vi "Interface.vi"(9 "EventsIn":T2, 10 "Events":T3) -> ()   [LabVIEW 2014, in "VIExecutionProperties.lvlib" / "VIExecutionProperties.lvclass"]
uses:
  VIExecutionProperties.lvclass
  Framework/_Plugins/_LVCMPlugin/GCMPlugin_EventsOut.ctl
  Framework/_Plugins/_LVCMPlugin/GCMPlugin_EventsIn.ctl
  Command.ctl
  Framework/_Plugins/GCMPlugin/GCMPlugin.lvclass
panel:
  out "LastCompiledWith":string caption="Last Compiled With:"
  out "CompiledCodeComplexity":dbl caption="Compiled Code Complexity:" format="%.0g"
  out "CodeSize":dbl caption="Code:" format="%01.1f kB"
  out "DataSize":dbl caption="Data:" format="%01.1f kB"
  out "BlockDiagramSize":dbl caption="Block Diagram:" format="%01.1f kB"
  out "FrontPanelSize":dbl caption="Front Panel:" format="%01.1f kB"
  in  "SuspendWhenCalled":bool caption="Suspend when called"
  in  "RunOnOpen":bool caption="Run when opened"
  in  "AutoErrHandling":bool caption="Enable auto error handling"
  in  "Priority":u16(ring) items=["invalid priority", "background", "normal", "above normal", "high", "time critical", "subroutine"]
  in  "PrefferedExecSystem":u16(ring) caption="Preffered execution system" items=["invalid execution system", "user interface", "standard", "instrument i/o", "data acquisition", "other 1", "other 2", "same as caller"]
  in  "Reentrancy":T1(radio)
  in  "InlineSubVI":bool caption="Inline subVI into calling VIs"
  in  "AllowDebugging":bool caption="Allow Debugging"
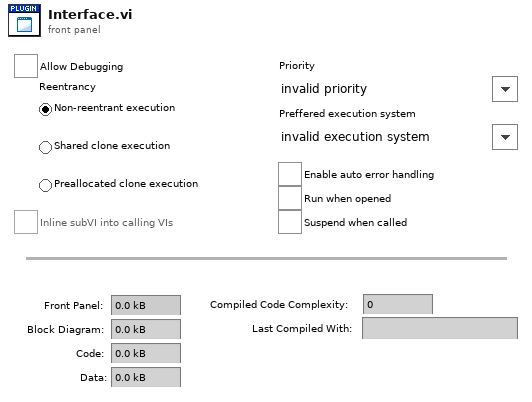
[diagram p1: front panel]
types:
  T1 = enum32{"Non-reentrant", "Shared clone", "Preallocated clone"}
  T2 = typedef "GCMPlugin.lvclass/GCMPlugin_EventsIn.ctl" = cluster{"Stop":refnum<user-event>, "ItemSelected":refnum<user-event>, "ItemDeselected":refnum<user-event>, "PluginActivated":refnum<user-event>, "PluginDeactivated":refnum<user-event>}
  T3 = typedef "GCMPlugin.lvclass/GCMPlugin_EventsOut.ctl" = cluster{"ItemEdited":refnum<user-event>}
  T4 = enum16{"Share clones between instances", "Preallocate clone for each instance"}
  T5 = enum8{"Enabled", "Disabled", "Disabled and Grayed Out"}
  T6 = typedef "VIExecutionProperties.lvlib/VIExecutionProperties.lvclass/Command.ctl" = enum16{"SaveVI", "LoadVIProperties", "Stop"}
  T7 = enum32{"invalid execution system", "user interface", "standard", "instrument i/o", "data acquisition", "other 1", "other 2", "same as caller"}
  T8 = enum32{"invalid priority", "background priority", "normal priority", "above normal priority", "high priority", "time critical priority", "subroutine"}
  T9 = typedef "LVLastCompiledWithTypeDef.ctl" = enum16{"Partial compiler optimizations", "Full compiler optimizations"}
  T10 = cluster{"Metric.FPSize":u32, "Metric.BDSize":u32, "Metric.CodeSize":u32, "Metric.DataSize":u32}
  T11 = cluster{"Metric.FPSize":dbl, "Metric.BDSize":dbl, "Metric.CodeSize":dbl, "Metric.DataSize":dbl}
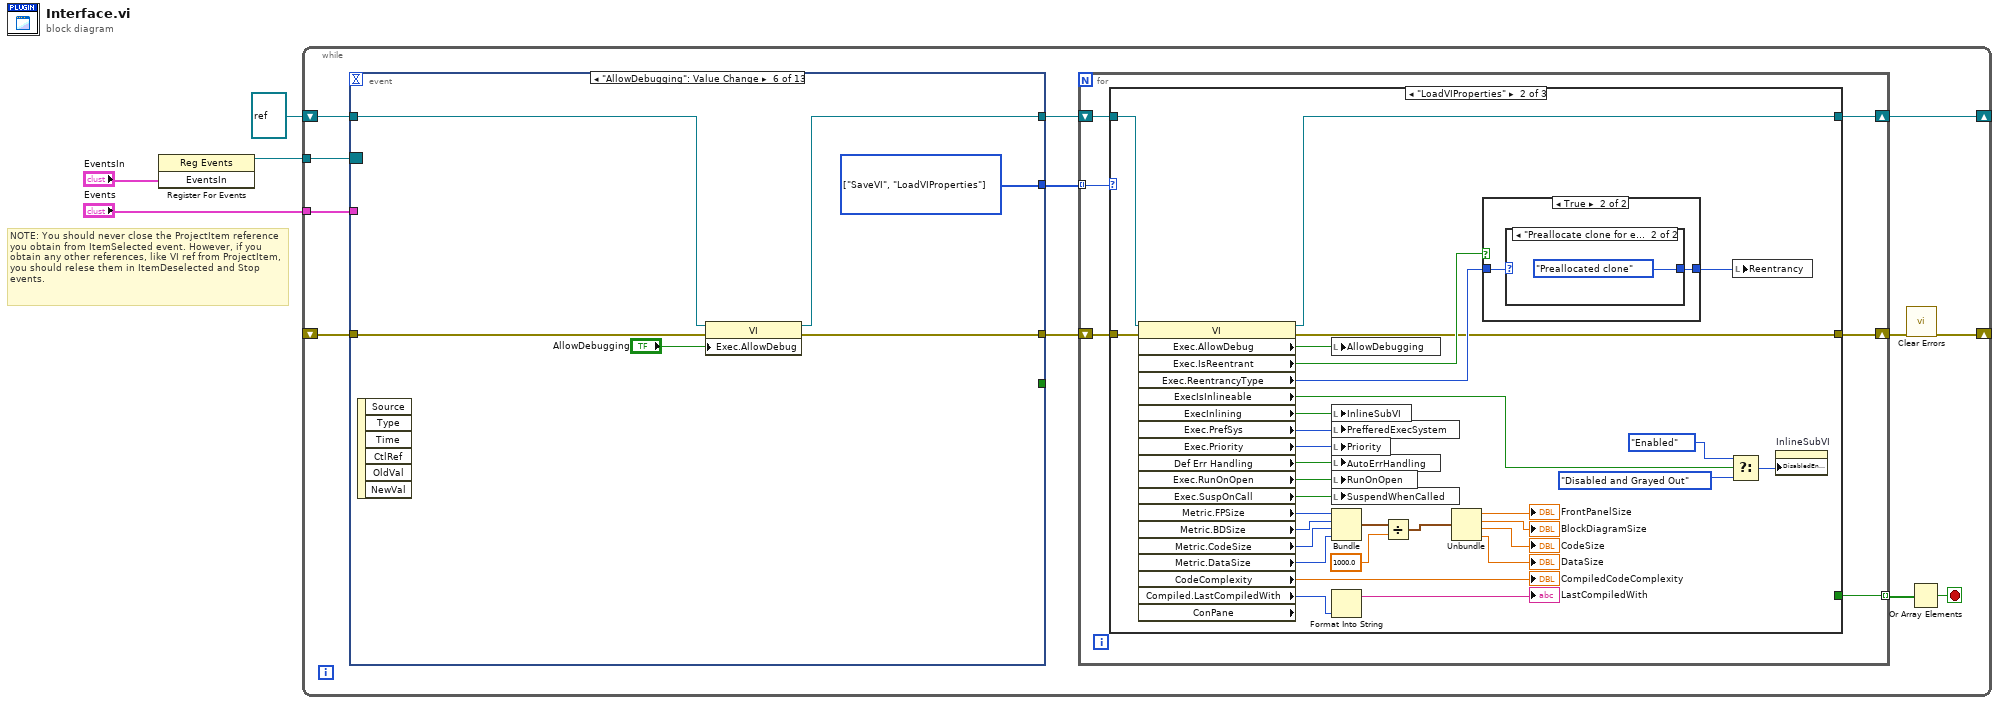
[diagram p0: block diagram]
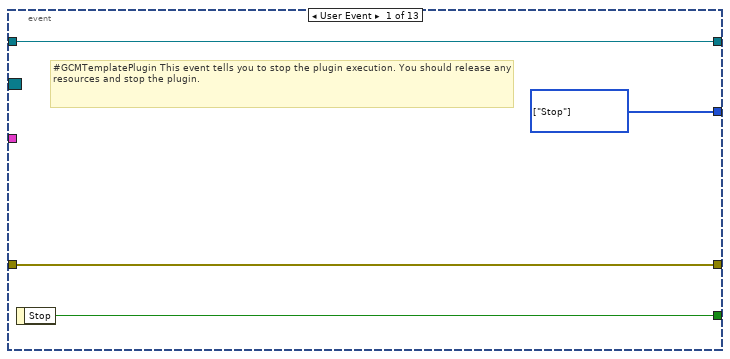
[diagram p2: hidden frame]
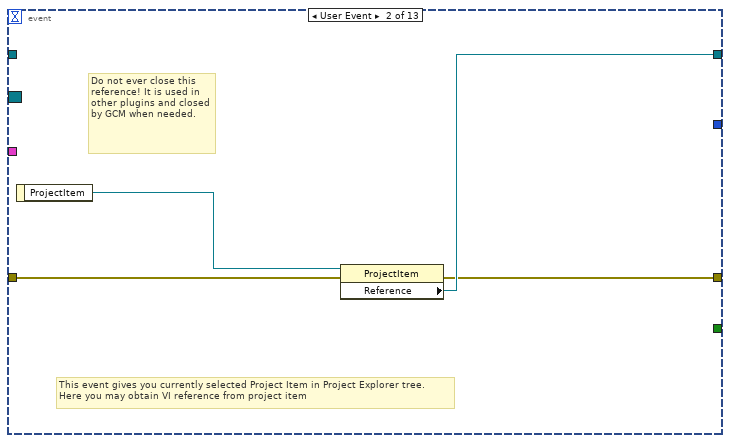
[diagram p3: hidden frame]
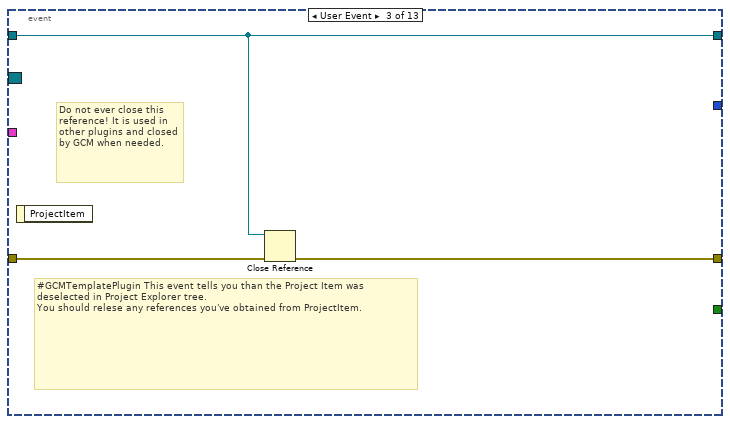
[diagram p4: hidden frame]
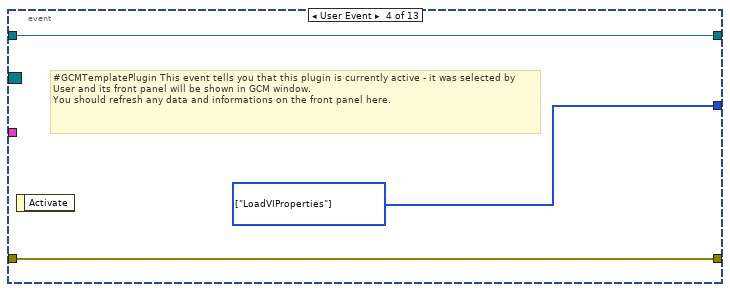
[diagram p5: hidden frame]
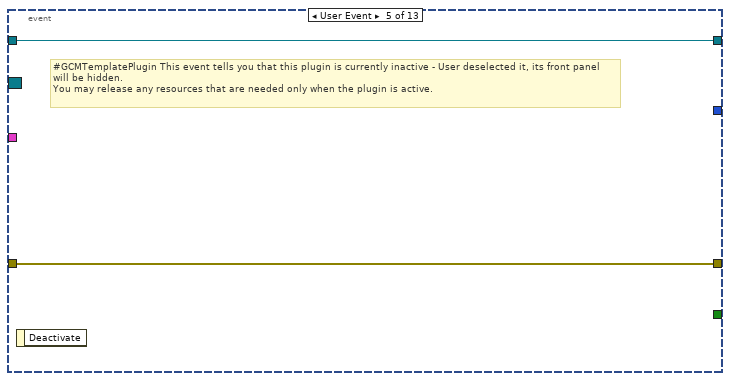
[diagram p6: hidden frame]
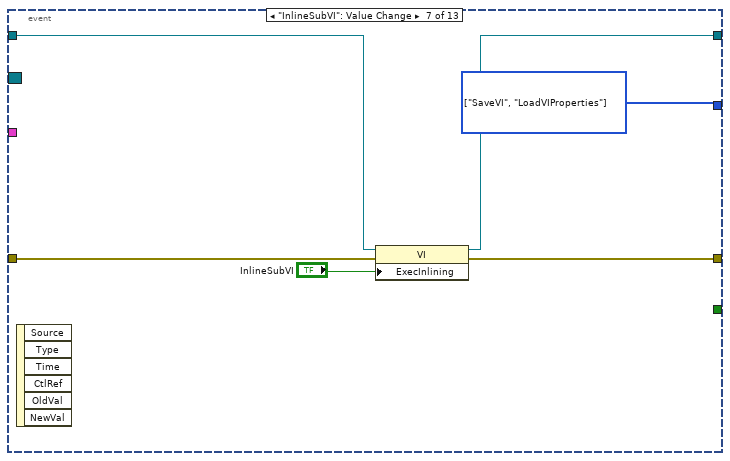
[diagram p7: hidden frame]
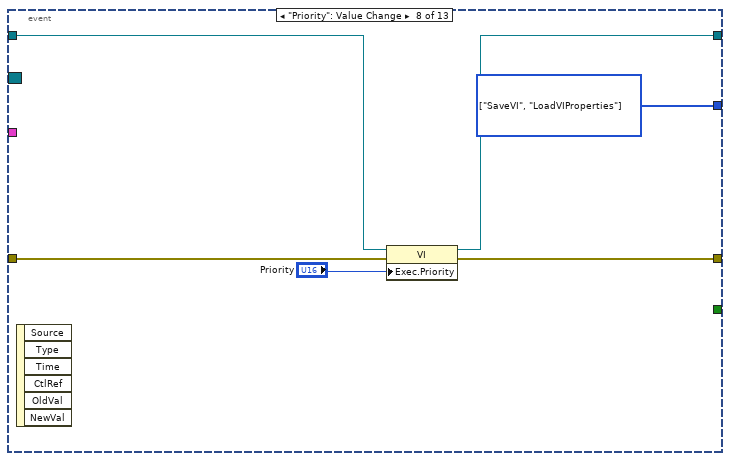
[diagram p8: hidden frame]
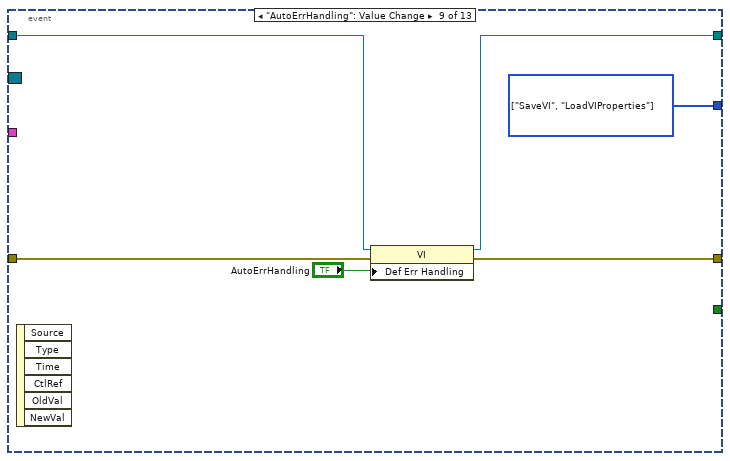
[diagram p9: hidden frame]
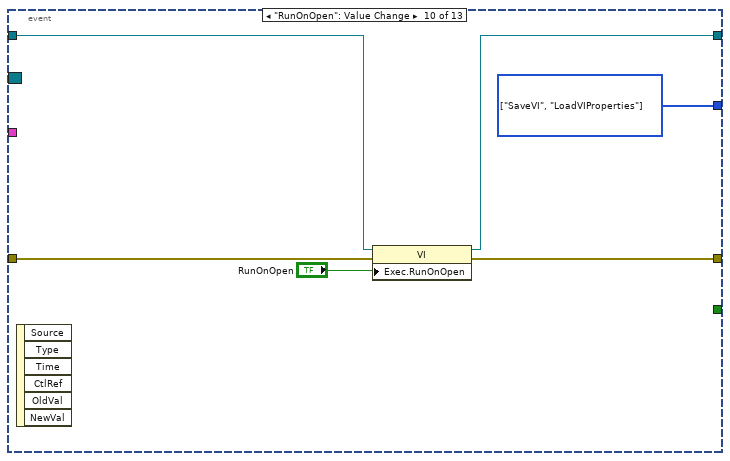
[diagram p10: hidden frame]
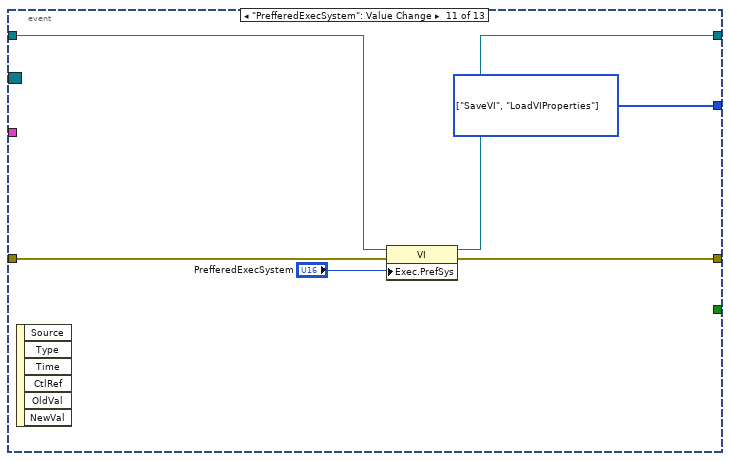
[diagram p11: hidden frame]
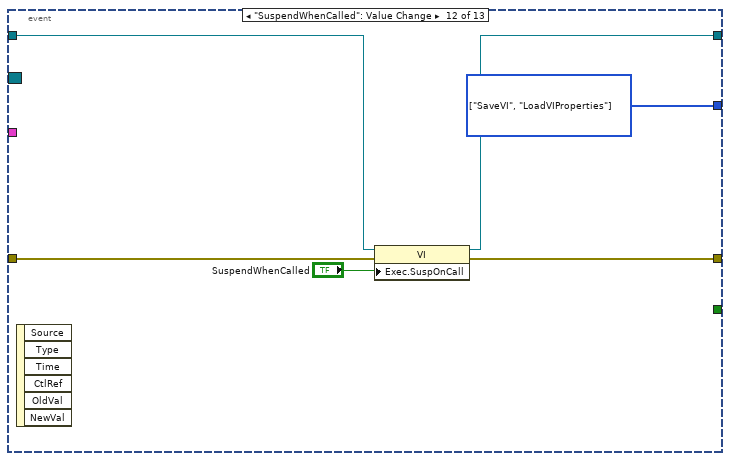
[diagram p12: hidden frame]
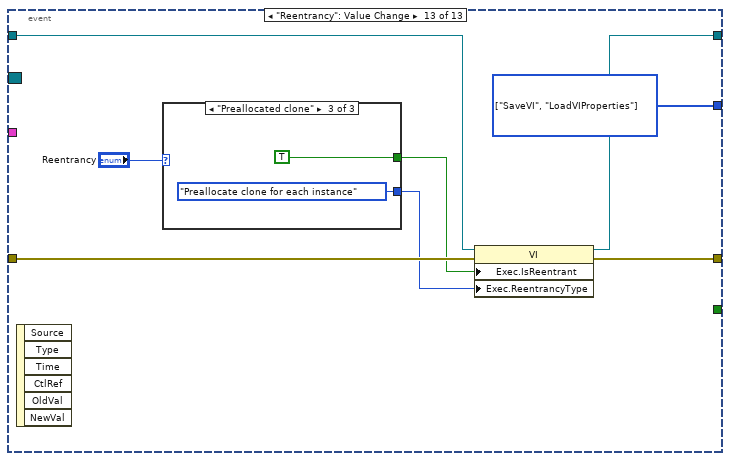
[diagram p13: hidden frame]
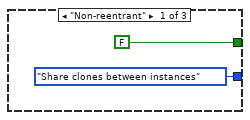
[diagram p14: hidden frame]
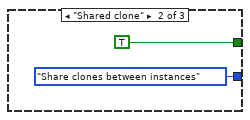
[diagram p15: hidden frame]
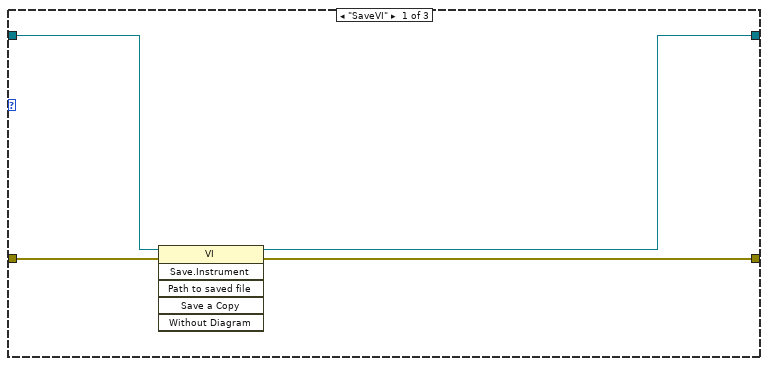
[diagram p16: hidden frame]
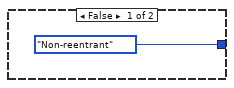
[diagram p17: hidden frame]
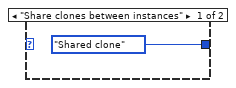
[diagram p18: hidden frame]
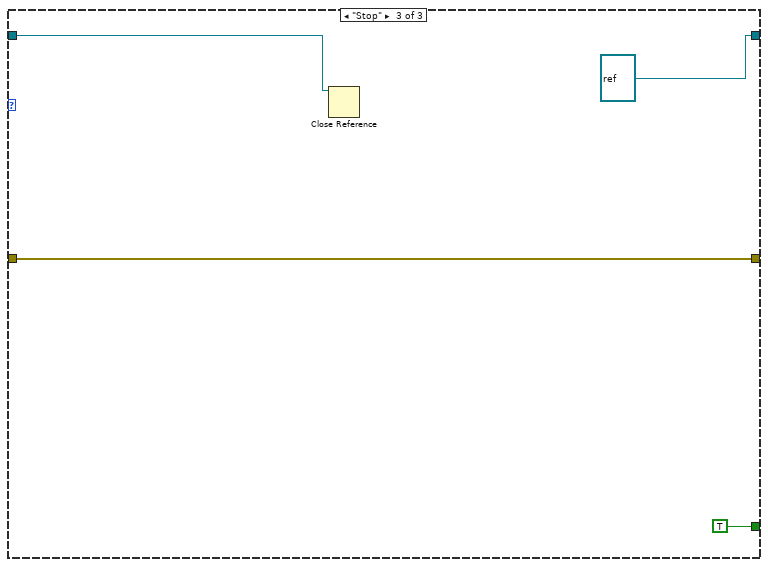
[diagram p19: hidden frame]
diagram:
  # "NOTE: You should never close the ProjectItem reference you obtain from ItemSelected event. However, if you obtain any other references, like VI ref from ProjectItem, you should relese them in ItemDeselected and Stop events."
  n1 = register-events("EventsIn") -> (reference out=w3:refnum<event-registration>)  [unwired: 2 in, 1 out]
  n2 = while {
    tunnel: w3 -> [w16]
    tunnel: "Events" -> [w15]
    shift-right: [w8] -> _
    shift-left: refnum<vi> refnum ("Reference") -> [w14]
    shift-right: [w11] -> _
    shift-left: _ -> [w12]
    stop <- w5 stop-if-true
    n3 = event shown="[5] \"AllowDebugging\": Value Change" {
      selector: w16 -> [_ _ _ _ _ _ _ _ _ _ _ _ _]
      dyn-events: _ -> [_ _ _ _ _ _ _ _ _ _ _ _ _]
      timeout: _ -> [_ _ _ _ _ _ _ _ _ _ _ _ _]
      tunnel: w15 -> [_ _ _ _ _ _ _ _ _ _ _ _ _]
      tunnel: [w20 _ _ _ _ _ _ _ _ _ _ _ _] -> _
      tunnel: [w19 w23 w27 w28 w32 w34 w41 w47 w53 w59 w65 w71 w79] -> w9
      tunnel: w14 -> [w19 _ w27 w28 w32 w35 w42 w48 w54 w60 w66 w72 w80]
      tunnel: [w18 w22 w25 w29 w31 w37 w43 w49 w55 w61 w67 w73 w81] -> w13
      tunnel: w12 -> [w18 w21 w26 w29 w31 w38 w44 w50 w56 w62 w68 w74 w82]
      tunnel: [w17 _ _ w30 _ w33 w39 w45 w51 w57 w63 w69 w75] -> w7
      event User Event {
        w17 = T6[] [enum."Stop"] items=["SaveVI", "LoadVIProperties", "Stop"]
        # "#GCMTemplatePlugin This event tells you to stop the plugin execution. You should release any resources and stop the plugin."
        n4 = event-data() -> ("Stop"=w20:bool)  [unwired: 1 in]
      }
      event User Event {
        # "Do not ever close this reference! It is used in other plugins and closed by GCM when needed."
        # "This event gives you currently selected Project Item in Project Explorer tree.\nHere you may obtain VI reference from project item"
        n5 = event-data() -> ("ProjectItem"=w24:refnum<vi>)  [unwired: 1 in]
        n6 = property class="ProjectItem"(reference=w24, error in=w21) -> (error out=w22:errorcluster, "Reference"=w23:refnum<vi>)  [unwired: 1 out]
      }
      event User Event {
        # "Do not ever close this reference! It is used in other plugins and closed by GCM when needed."
        # "#GCMTemplatePlugin This event tells you than the Project Item was deselected in Project Explorer tree.\nYou should relese any references you've obtained from ProjectItem."
        n7 = event-data() -> ()  [unwired: 1 in, 1 out]
        n8 = Close Reference(reference=w27, error in (no error)=w26) -> (error out=w25:errorcluster)
      }
      event User Event {
        w30 = T6[] [enum."LoadVIProperties"] items=["SaveVI", "LoadVIProperties", "Stop"]
        # "#GCMTemplatePlugin This event tells you that this plugin is currently active - it was selected by User and its front panel will be shown in GCM window.\nYou should refresh any data and informations on the front panel here."
        n9 = event-data() -> ()  [unwired: 1 in, 1 out]
      }
      event User Event {
        # "#GCMTemplatePlugin This event tells you that this plugin is currently inactive - User deselected it, its front panel will be hidden.\nYou may release any resources that are needed only when the plugin is active."
        n10 = event-data() -> ()  [unwired: 1 in, 1 out]
      }
      event "AllowDebugging": Value Change {
        w33 = T6[] [enum."SaveVI", enum."LoadVIProperties"] items=["SaveVI", "LoadVIProperties", "Stop"]
        n11 = event-data() -> ()  [unwired: 1 in, 6 out]
        n12 = property class="VI"(reference=w35, error in=w38, "Exec.AllowDebug"="AllowDebugging") -> (reference out=w34:refnum<vi>, error out=w37:errorcluster)
      }
      event "InlineSubVI": Value Change {
        w39 = T6[] [enum."SaveVI", enum."LoadVIProperties"] items=["SaveVI", "LoadVIProperties", "Stop"]
        n13 = event-data() -> ()  [unwired: 1 in, 6 out]
        n14 = property class="VI"(reference=w42, error in=w44, "ExecInlining"="InlineSubVI") -> (reference out=w41:refnum<vi>, error out=w43:errorcluster)
      }
      event "Priority": Value Change {
        w45 = T6[] [enum."SaveVI", enum."LoadVIProperties"] items=["SaveVI", "LoadVIProperties", "Stop"]
        n15 = event-data() -> ()  [unwired: 1 in, 6 out]
        n16 = property class="VI"(reference=w48, error in=w50, "Exec.Priority"="Priority") -> (reference out=w47:refnum<vi>, error out=w49:errorcluster)
      }
      event "AutoErrHandling": Value Change {
        w51 = T6[] [enum."SaveVI", enum."LoadVIProperties"] items=["SaveVI", "LoadVIProperties", "Stop"]
        n17 = event-data() -> ()  [unwired: 1 in, 6 out]
        n18 = property class="VI"(reference=w54, error in=w56, "Def Err Handling"="AutoErrHandling") -> (reference out=w53:refnum<vi>, error out=w55:errorcluster)
      }
      event "RunOnOpen": Value Change {
        w57 = T6[] [enum."SaveVI", enum."LoadVIProperties"] items=["SaveVI", "LoadVIProperties", "Stop"]
        n19 = event-data() -> ()  [unwired: 1 in, 6 out]
        n20 = property class="VI"(reference=w60, error in=w62, "Exec.RunOnOpen"="RunOnOpen") -> (reference out=w59:refnum<vi>, error out=w61:errorcluster)
      }
      event "PrefferedExecSystem": Value Change {
        w63 = T6[] [enum."SaveVI", enum."LoadVIProperties"] items=["SaveVI", "LoadVIProperties", "Stop"]
        n21 = event-data() -> ()  [unwired: 1 in, 6 out]
        n22 = property class="VI"(reference=w66, error in=w68, "Exec.PrefSys"="PrefferedExecSystem") -> (reference out=w65:refnum<vi>, error out=w67:errorcluster)
      }
      event "SuspendWhenCalled": Value Change {
        w69 = T6[] [enum."SaveVI", enum."LoadVIProperties"] items=["SaveVI", "LoadVIProperties", "Stop"]
        n23 = event-data() -> ()  [unwired: 1 in, 6 out]
        n24 = property class="VI"(reference=w72, error in=w74, "Exec.SuspOnCall"="SuspendWhenCalled") -> (reference out=w71:refnum<vi>, error out=w73:errorcluster)
      }
      event "Reentrancy": Value Change {
        w75 = T6[] [enum."SaveVI", enum."LoadVIProperties"] items=["SaveVI", "LoadVIProperties", "Stop"]
        n25 = event-data() -> ()  [unwired: 1 in, 6 out]
        n26 = case shown="\"Preallocated clone\"" "Reentrancy" {
          tunnel: [FALSE ("Execution:Is Reentrant") TRUE ("Execution:Is Reentrant") TRUE ("Execution:Is Reentrant")] -> w77
          tunnel: [T4."Share clones between instances" ("Execution:Reentrancy Type") T4."Share clones between instances" ("Execution:Reentrancy Type") T4."Preallocate clone for each instance" ("Execution:Reentrancy Type")] -> w76
          frame "Non-reentrant" {
          }
          frame "Shared clone" {
          }
          frame "Preallocated clone" {
          }
        }
        n27 = property class="VI"(reference=w80, error in=w82, "Exec.IsReentrant"=w77, "Exec.ReentrancyType"=w76) -> (reference out=w79:refnum<vi>, error out=w81:errorcluster)
      }
    }
    n28 = for {
      shift-right: [w93] -> w10
      shift-left: w13 -> [w94]
      shift-right: [w91] -> w8
      shift-left: w9 -> [w92]
      tunnel: w7 -> [w90] mode=indexing
      tunnel: [w89] -> w6 mode=indexing
      n29 = case shown="\"LoadVIProperties\"" w90 {
        tunnel: w94 -> [w98 w102 w139]
        tunnel: [w97 w99 w139] -> w93
        tunnel: w92 -> [w96 w101 w137]
        tunnel: [w95 w100 refnum<vi> refnum ("Reference")] -> w91
        tunnel: [_ _ TRUE] -> w89
        frame "SaveVI" {
          n30 = invoke class="VI" method="Save.Instrument"(reference=w96, error in=w98) -> (reference out=w95:refnum<vi>, error out=w97:errorcluster)  [unwired: 4 in, 4 out]
        }
        frame "LoadVIProperties" {
          n31 = property class="VI" props=["Exec.AllowDebug", "Exec.IsReentrant", "Exec.ReentrancyType", "ExecIsInlineable", "ExecInlining", "Exec.PrefSys", "Exec.Priority", "Def Err Handling", "Exec.RunOnOpen", "Exec.SuspOnCall", "Metric.FPSize", "Metric.BDSize", "Metric.CodeSize", "Metric.DataSize", "CodeComplexity", "Compiled.LastCompiledWith", "ConPane"](reference=w101, error in=w102) -> (reference out=w100:refnum<vi>, error out=w99:errorcluster, "Exec.AllowDebug"=w103:bool, "Exec.IsReentrant"=w107:bool, "Exec.ReentrancyType"=w108:T4, "ExecIsInlineable"=w130:bool, "ExecInlining"=w104:bool, "Exec.PrefSys"=w106:T7, "Exec.Priority"=w105:T8, "Def Err Handling"=w110:bool, "Exec.RunOnOpen"=w112:bool, "Exec.SuspOnCall"=w111:bool, "Metric.FPSize"=w113:u32, "Metric.BDSize"=w117:u32, "Metric.CodeSize"=w118:u32, "Metric.DataSize"=w119:u32, "CodeComplexity"=→"CompiledCodeComplexity":sgl, "Compiled.LastCompiledWith"=w115:T9)  [unwired: 1 out]
          n32 = local write "AllowDebugging"(w103) -> ()
          n33 = local write "InlineSubVI"(w104) -> ()
          n34 = local write "PrefferedExecSystem"(w106) -> ()
          n35 = local write "Priority"(w105) -> ()
          n36 = local write "AutoErrHandling"(w110) -> ()
          n37 = local write "RunOnOpen"(w112) -> ()
          n38 = local write "SuspendWhenCalled"(w111) -> ()
          n39 = Bundle("Metric.FPSize"=w113, "Metric.BDSize"=w117, "Metric.CodeSize"=w118, "Metric.DataSize"=w119) -> (w120:T10)  [unwired: 1 in]
          n40 = Format Into String(w115) -> (resulting string=→"LastCompiledWith":string)  [unwired: 3 in, 1 out]
          n41 = Divide(x=w120, y=1000.0) -> (x/y=w122:T11)
          n42 = Unbundle(w122) -> ("Metric.FPSize"=→"FrontPanelSize":dbl, "Metric.BDSize"=→"BlockDiagramSize":dbl, "Metric.CodeSize"=→"CodeSize":dbl, "Metric.DataSize"=→"DataSize":dbl)
          n43 = case shown="True" w107 {
            tunnel: w108 -> [_ w133]
            tunnel: [T1."Non-reentrant" ("Reentrancy") w132] -> w109
            frame False {
            }
            frame True {
              n44 = case shown="\"Preallocate clone for each instance\"" w133 {
                tunnel: [T1."Shared clone" ("Reentrancy") T1."Preallocated clone" ("Reentrancy")] -> w132
                frame "Share clones between instances" {
                }
                frame "Preallocate clone for each instance" {
                }
              }
            }
          }
          n45 = Select(t=T5."Enabled" ("Disabled"), s=w130, f=T5."Disabled and Grayed Out") -> (s? t:f=w128:T5)
          n46 = local write "Reentrancy"(w109) -> ()
          n47 = property on="InlineSubVI" class="Bool (strict)"("DisabledEnum"=w128) -> ()  [unwired: 2 in, 2 out]
        }
        frame "Stop" {
          n48 = Close Reference(reference=w137) -> ()  [unwired: 1 in, 1 out]
        }
      }
    }
    n49 = call <vilib>:"Clear Errors.vi"("error in (no error)"=w10) -> ("error out"=w11:errorcluster)  [unwired: 5 in, 1 out]
    n50 = Or Array Elements(Boolean array=w6) -> (logical OR=w5:bool)
  }
